vi "Voltage -Output.vi"(8 "Entrada de erro":errorcluster, 9 "Onda":waveform(dbl)={"t0"=timestamp(0 s since 1904-01-01), "dt"=0.0, "Y"=[]}, 10 "Canal físico":tag, 11 "Task/Canal entrada":refnum<k21>) -> (0 "Saída de erro":errorcluster)   [LabVIEW 2020]
doc: "This example demonstrates how to continuously re-generate analog output data from a buffer in your computer's memory.\n\nRefer to your device documentation for pinouts and hardware capabilities."
uses:
  <vilib>/DAQmx/miscellaneous.llb/DAQmx Fill In Error Info.vi
  <vilib>/DAQmx/write.llb/DAQmx Write (Analog Wfm 1Chan NSamp).vi
  <vilib>/DAQmx/create/channels.llb/DAQmx Create Channel (AO-Voltage-Basic).vi
  <vilib>/DAQmx/configure/timing.llb/DAQmx Timing (Sample Clock).vi
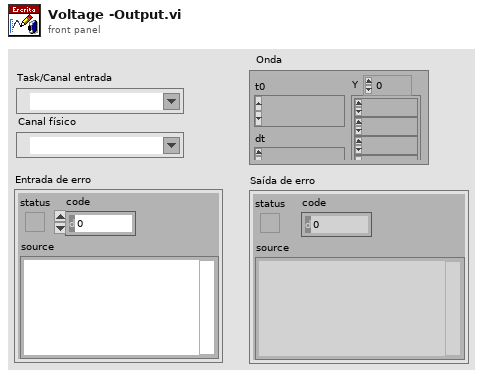
[diagram p1: front panel]
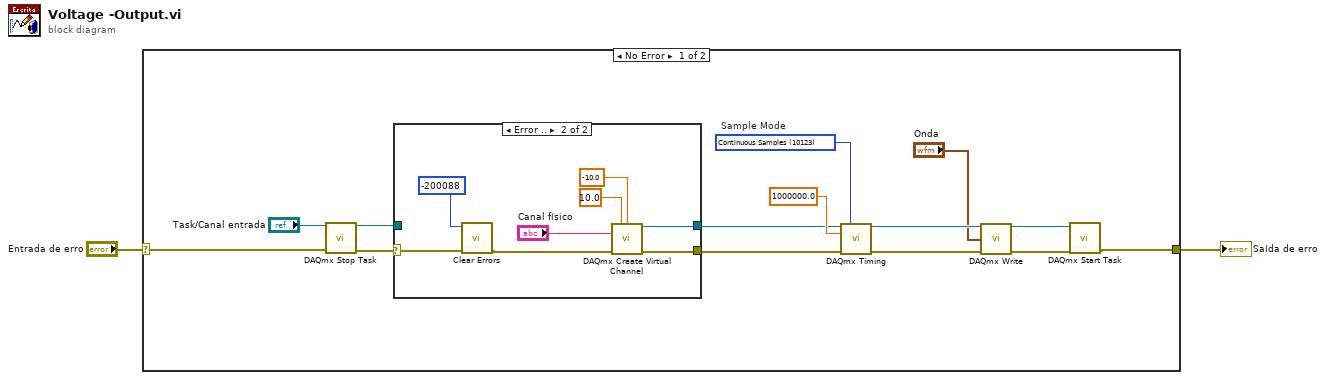
[diagram p0: block diagram]
diagram:
  n1 = case shown="No Error" "Entrada de erro" {
    selector: "Entrada de erro" -> [w5 w27]
    tunnel: [w4 w27] -> w2
    frame No Error {
      w16 = 10123 items=["Finite Samples"=10178, "Continuous Samples"=10123, "Hardware Timed Single Point"=12522]  # Sample Mode
      n2 = call <vilib>:"DAQmx Stop Task.vi"("task/channels in"="Task/Canal entrada", "error in"=w5) -> ("task out"=w10:refnum<k21>, "error out"=w11:errorcluster)  [unwired: 12 in]
      n3 = case shown="Error .." w11 {
        selector: w11 -> [w18 w26]
        tunnel: [w18 w20] -> w9
        tunnel: [w17 w21] -> w8
        tunnel: w10 -> [w17 _]
        frame No Error {
        }
        frame Error {
          n4 = call <vilib>:"Clear Errors.vi"("error in (no error)"=w26, "specific error code to clear (0: all)"=-200088) -> ("error out"=w22:errorcluster)  [unwired: 4 in, 1 out]
          n5 = call-poly <vilib>:"DAQmx Create Virtual Channel.vi"("maximum value"=10.0, "minimum value"=-10.0, "physical channels"="Canal físico", "error in"=w22) -> ("task out"=w21:refnum<k21>, "error out"=w20:errorcluster)  [unwired: 10 in]
        }
      }
      n6 = call-poly <vilib>:"DAQmx Timing.vi"("task/channels in"=w8, "sample mode"=w16, "rate"=1000000.0, "error in"=w9) -> ("task out"=w13:refnum<k21>, "error out"=w6:errorcluster)  [unwired: 10 in]
      n7 = call-poly <vilib>:"DAQmx Write.vi"("task/channels in"=w13, "data"="Onda", "error in"=w6) -> ("task out"=w15:refnum<k21>, "error out"=w14:errorcluster)  [unwired: 10 in, 1 out]
      n8 = call <vilib>:"DAQmx Start Task.vi"("task/channels in"=w15, "error in"=w14) -> ("error out"=w4:errorcluster)  [unwired: 12 in, 1 out]
    }
    frame Error {
    }
  }
  "Saída de erro" <- w2
